vi "Convert Data Bytes to HW number.vi"(11 "Bytes":u8[](array[numeric]) format="%.0x") -> (3 "HW part number":string)   [LabVIEW 2023]
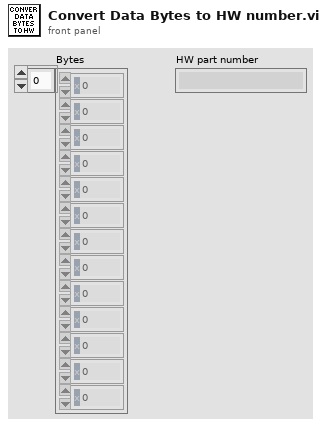
[diagram p1: front panel]
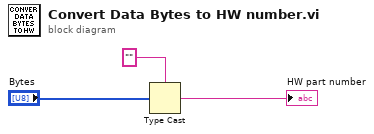
[diagram p0: block diagram]
diagram:
  n1 = Type Cast(type="" ("HW part number"), x="Bytes") -> (*(type *) &x=→"HW part number":string)
